vi "Get PMU Real Data.vi"(5 "Action":enum16{"Initialize", "Read", "Reset"}(ring)=enum."Read", 7 "PMU Configuration":T2(array[cluster]), 10 "PMU Index":i32, 11 "Pseudo PDC ID":i32) -> (2 "PMU Data":T3, 3 "Data OK":bool, 4 "status":T1)   [LabVIEW 2013, in "PMU Recorder Light.lvlib" / "Statnett C37.118 DLL.lvclass"]
uses:
  Statnett C37.118 DLL.lvclass
  c37118-dll/labview/C37118-DLL.lvlib
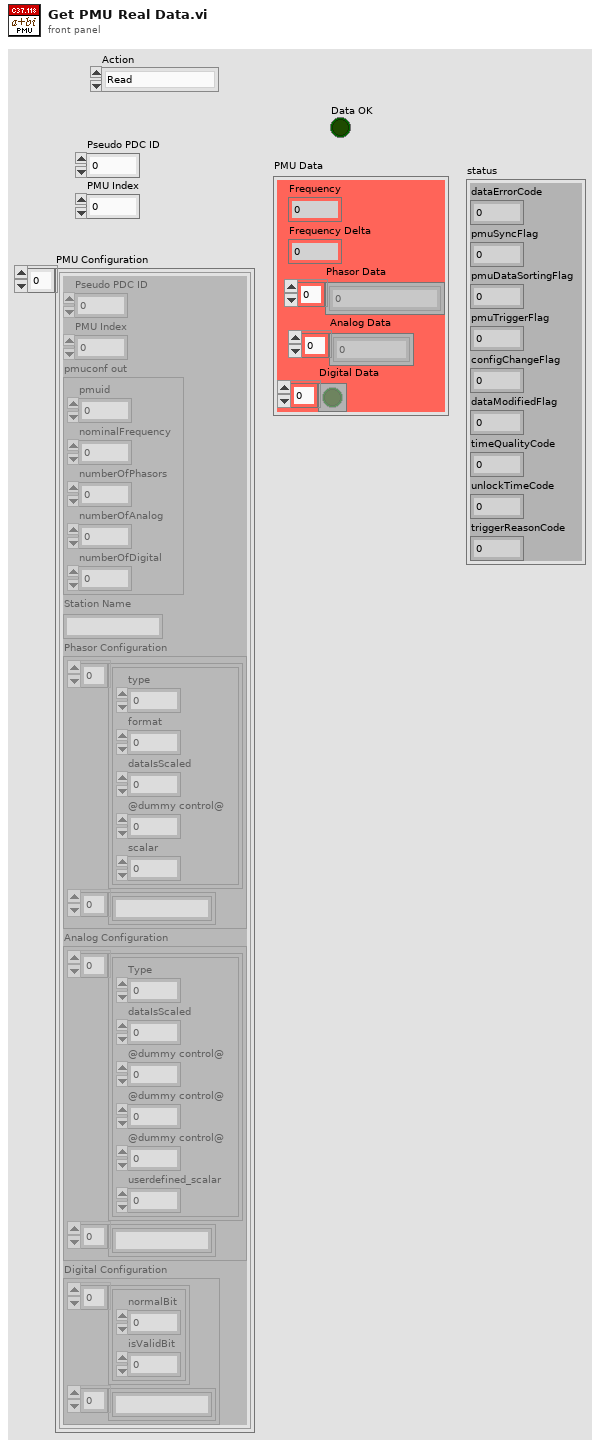
[diagram p1: front panel]
types:
  T1 = cluster{"dataErrorCode":u8, "pmuSyncFlag":u8, "pmuDataSortingFlag":u8, "pmuTriggerFlag":u8, "configChangeFlag":u8, "dataModifiedFlag":u8, "timeQualityCode":u8, "unlockTimeCode":u8, "triggerReasonCode":u8}
  T2 = cluster{"Pseudo PDC ID":i32, "PMU Index":i32, "pmuconf out":cluster{"pmuid":i32, "nominalFrequency":sgl, "numberOfPhasors":i32, "numberOfAnalog":i32, "numberOfDigital":i32}, "Station Name":string, "Phasor Configuration":cluster{cluster{"type":u8, "format":u8, "dataIsScaled":u8, "@dummy control@":i8, "scalar":sgl}[], string[]}, "Analog Configuration":cluster{cluster{"Type":i32, "dataIsScaled":u8, "@dummy control@":i8, "@dummy control@":i8, "@dummy control@":i8, "userdefined_scalar":sgl}[], string[]}, "Digital Configuration":cluster{cluster{"normalBit":u8, "isValidBit":u8}[], string[]}}[]
  T3 = cluster{"Frequency":sgl, "Frequency Delta":sgl, "Phasor Data":csg[], "Analog Data":sgl[], "Digital Data":bool[]}
  T4 = cluster{"Array Lengths":cluster{"Phasor":i32, "Analog":i32, "Digital":i32}, "Phasor Scaling":cluster{"Format":bool[], "Data Is Scaled":bool[], "Scaling":sgl[]}, "Analog Scaling":cluster{"Data Is Scaled":bool[], "Scaling":sgl[]}}
  T5 = cluster{cluster{"type":u8, "format":u8, "dataIsScaled":u8, "@dummy control@":i8, "scalar":sgl}[], string[]}
  T6 = cluster{cluster{"Type":i32, "dataIsScaled":u8, "@dummy control@":i8, "@dummy control@":i8, "@dummy control@":i8, "userdefined_scalar":sgl}[], string[]}
  T7 = cluster{"Rectangular(T)/Polar(F)":bool[], "Data Is Scaled":bool[], "Scaling":sgl[]}
  T8 = cluster{"Data Is Scaled":bool[], "Scaling":sgl[]}
  T9 = cluster{"Array Lengths":cluster{"Phasor":i32, "Analog":i32, "Digital":i32}, "Phasor Scaling":cluster{"Format":bool[], "Data Is Scaled":bool[], "Scaling":sgl[]}, "Analog Scaling":cluster{"Data Is Scaled":bool[], "Scaling":sgl[]}}[]
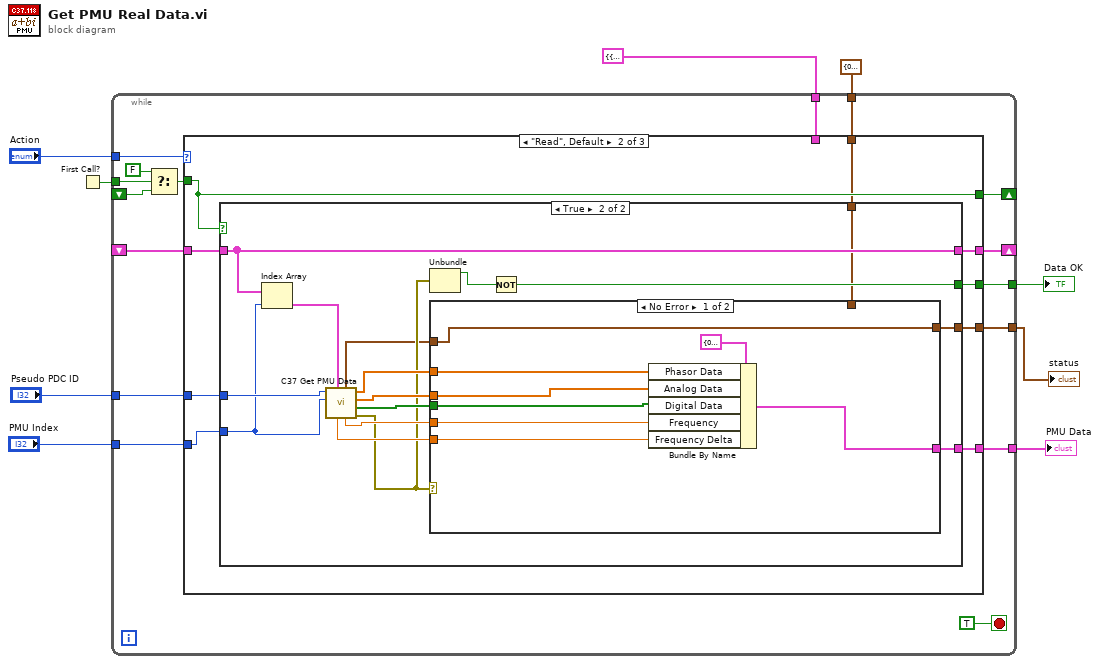
[diagram p0: block diagram]
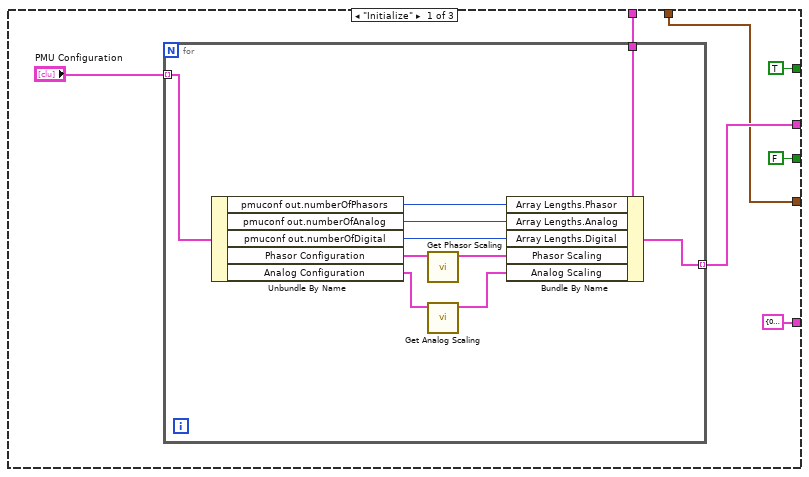
[diagram p2: hidden frame]
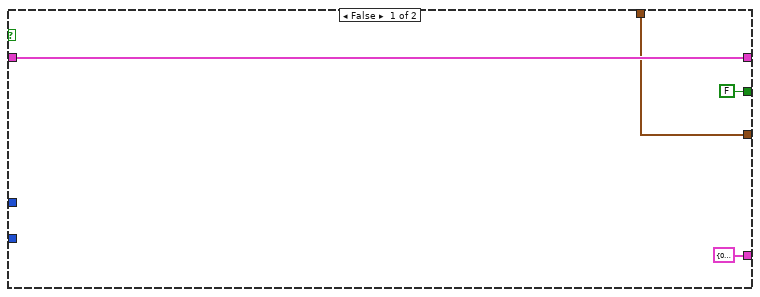
[diagram p3: hidden frame]
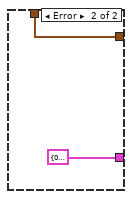
[diagram p4: hidden frame]
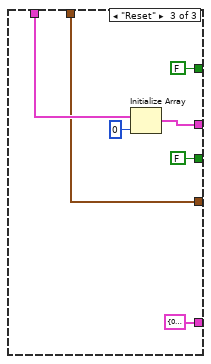
[diagram p5: hidden frame]
diagram:
  n1 = First Call?() -> (First Call?: T/F=w4:bool)
  n2 = while {
    tunnel: "Pseudo PDC ID" -> [w25]
    tunnel: "PMU Index" -> [w24]
    tunnel: [w23] -> w7
    tunnel: [w22] -> w6
    tunnel: "Action" -> [w20]
    shift-right: [w15] -> _
    shift-left: _ -> [w18]
    tunnel: w4 -> [w19]
    shift-right: [w13] -> _
    shift-left: _ -> [w14]
    tunnel: T4 {"Array Lengths"={"Phasor"=0, "Analog"=0, "Digital"=0}, "Phasor Scaling"={"Format"=[], "Data Is Scaled"=[], "Scaling"=[]}, "Analog Scaling"={"Data Is Scaled"=[], "Scaling"=[]}} ("Channel Info") -> [w12]
    tunnel: [w11] -> w2
    tunnel: T1 {"dataErrorCode"=0, "pmuSyncFlag"=0, "pmuDataSortingFlag"=0, "pmuTriggerFlag"=0, "configChangeFlag"=0, "dataModifiedFlag"=0, "timeQualityCode"=0, "unlockTimeCode"=0, "triggerReasonCode"=0} ("status") -> [w10]
    stop <- TRUE stop-if-true
    n3 = Select(t=FALSE ("First Call?: T/F"), s=w19, f=w18) -> (s? t:f=w16:bool)
    n4 = case shown="\"Read\", Default" w20 {
      tunnel: w25 -> [_ w51 _]
      tunnel: w24 -> [_ w50 _]
      tunnel: [FALSE w49 FALSE] -> w23
      tunnel: [T3 {"Frequency"=0.0, "Frequency Delta"=0.0, "Phasor Data"=[], "Analog Data"=[], "Digital Data"=[]} ("PMU Data") w48 T3 {"Frequency"=0.0, "Frequency Delta"=0.0, "Phasor Data"=[], "Analog Data"=[], "Digital Data"=[]} ("PMU Data")] -> w22
      tunnel: w16 -> [_ w47 _]
      tunnel: [TRUE ("First Call?: T/F") w47 FALSE ("First Call?: T/F")] -> w15
      tunnel: w14 -> [_ w46 _]
      tunnel: [w32 w45 w83] -> w13
      tunnel: w12 -> [w27 _ w85]
      tunnel: [w26 w44 w82] -> w11
      tunnel: w10 -> [w26 w43 w82]
      frame "Initialize" {
        n5 = for {
          tunnel: [w42] -> w32 mode=indexing
          tunnel: "PMU Configuration" -> [w41] mode=indexing
          tunnel: w27 -> [w33]
          n6 = Unbundle By Name(w41) -> ("pmuconf out.numberOfPhasors"=w40:i32, "pmuconf out.numberOfAnalog"=w39:i32, "pmuconf out.numberOfDigital"=w38:i32, "Phasor Configuration"=w37:T5, "Analog Configuration"=w36:T6)
          n7 = call "Get Phasor Scaling.vi"("Phasor Configuration"=w37) -> ("Phasor Scaling"=w34:T7)  [unwired: 10 in]
          n8 = call "Get Analog Scaling.vi"("Analog Configuration"=w36) -> ("Analog Scaling"=w35:T8)  [unwired: 10 in]
          n9 = Bundle By Name(cluster=w33, "Array Lengths.Phasor"=w40, "Array Lengths.Analog"=w39, "Array Lengths.Digital"=w38, "Phasor Scaling"=w34, "Analog Scaling"=w35) -> (w42:T4)
        }
      }
      frame "Read", Default {
        n10 = case shown="True" w47 {
          tunnel: w51 -> [_ w69]
          tunnel: w50 -> [_ w68]
          tunnel: [FALSE w59] -> w49
          tunnel: [T3 {"Frequency"=0.0, "Frequency Delta"=0.0, "Phasor Data"=[], "Analog Data"=[], "Digital Data"=[]} ("PMU Data") w71] -> w48
          tunnel: w46 -> [w55 w70]
          tunnel: [w55 w70] -> w45
          tunnel: [w52 w57] -> w44
          tunnel: w43 -> [w52 w56]
          frame False {
          }
          frame True {
            n11 = Index Array(array=w70, index=w68) -> (element=w62:T4)
            n12 = call "C37 Get PMU Data.vi"("Channel Info"=w62, "PMU Index"=w68, "Pseudo PDC ID"=w69) -> ("error out"=w61:errorcluster, "Digital Values"=w65:bool[], "Analog Values"=w66:sgl[], "Phasor Values"=w67:csg[], "Frequency"=w64:sgl, "status"=w58:T1, "Delta Frequency"=w63:sgl)  [unwired: 2 in]
            n13 = Unbundle(w61) -> ("status"=w60:bool)  [unwired: 2 out]
            n14 = case shown="No Error" w61 {
              tunnel: [w79 T3 {"Frequency"=0.0, "Frequency Delta"=0.0, "Phasor Data"=[], "Analog Data"=[], "Digital Data"=[]} ("PMU Data")] -> w71
              tunnel: w67 -> [w78 _]
              tunnel: w66 -> [w77 _]
              tunnel: w65 -> [w76 _]
              tunnel: w64 -> [w75 _]
              tunnel: w63 -> [w74 _]
              tunnel: w58 -> [w72 _]
              tunnel: [w72 w80] -> w57
              tunnel: w56 -> [_ w80]
              frame No Error {
                n15 = Bundle By Name(cluster=T3 {"Frequency"=0.0, "Frequency Delta"=0.0, "Phasor Data"=[], "Analog Data"=[], "Digital Data"=[]} ("PMU Data"), "Phasor Data"=w78, "Analog Data"=w77, "Digital Data"=w76, "Frequency"=w75, "Frequency Delta"=w74) -> (w79:T3)
              }
              frame Error {
              }
            }
            n16 = Not(x=w60) -> (.not. x?=w59:bool)
          }
        }
      }
      frame "Reset" {
        n17 = Initialize Array(w85, 0 ("dimension size")) -> (w83:T9)
      }
    }
  }
  "PMU Data" <- w6
  "Data OK" <- w7
  "status" <- w2
